vi "AddStringToPath.vi"(9 "delimiter (/)":string="/", 10 "String":string, 11 "Path In":path) -> (3 "Path Out":path)   [LabVIEW 2016, in "NI_NPW_Loading Project Info.lvlib"]
uses:
  <resource>/dialog/NewProjectWizard/Loading Project Info/NI_NPW_Loading Project Info.lvlib
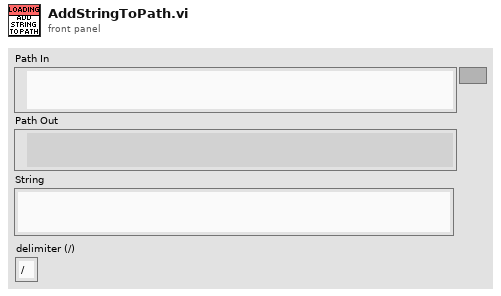
[diagram p1: front panel]
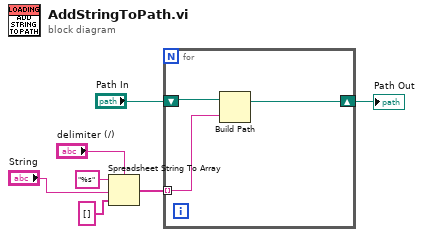
[diagram p0: block diagram]
diagram:
  n1 = Spreadsheet String To Array(delimiter (Tab)="delimiter (/)", format string="%s", spreadsheet string="String", array type (2D Dbl)=string[] []) -> (array=w2:string[])
  n2 = for {
    tunnel: w2 -> [w9] mode=indexing
    shift-right: [w8] -> w1
    shift-left: "Path In" -> [w10]
    n3 = Build Path(base path=w10, name or relative path=w9) -> (appended path=w8:path)
  }
  "Path Out" <- w1
